vi "LS_SETP.vi"(8 "error in (no error)":errorcluster, 9 "Set Point (K)":dbl, 10 "Data Cluster In":T3 {"GUI Data Cluster"."SBR" format="%08b"}, 11 "Config Cluster In":T1={"General"={"Config.ini"=path "", "Default Logging Path"=path ""}, "Hardware"={"Measure Rate (1/s)"=0, "HP DMM VISA"="", "LS 335 VISA"="", "HP DM"={"Range"=enum."Autorange", "Autozero"=FALSE, "Display"=enum."3 1/2 Digit", "Blank LCD"=FALSE}, "LS335"={"Brightness"=enum."25%"}}, "Operation"={"Operation Mode"=enum."Logging", "Status"="", "NewLog?"=FALSE, "OvenWarn"=FALSE, "LS335"={"Heater A"={"Range"=enum."Off", "Set Point"=0.0}, "Heater B"={"Range"=enum."Off", "Set Point"=0.0}}}}) -> (0 "error out":errorcluster, 2 "Data Cluster Out":T3 {"GUI Data Cluster"."SBR" format="%08b"}, 3 "Config Cluster Out":T1={"General"={"Config.ini"=path "", "Default Logging Path"=path ""}, "Hardware"={"Measure Rate (1/s)"=0, "HP DMM VISA"="", "LS 335 VISA"="", "HP DM"={"Range"=enum."Autorange", "Autozero"=FALSE, "Display"=enum."3 1/2 Digit", "Blank LCD"=FALSE}, "LS335"={"Brightness"=enum."25%"}}, "Operation"={"Operation Mode"=enum."Idle-Off", "Status"="", "NewLog?"=FALSE, "OvenWarn"=FALSE, "LS335"={"Heater A"={"Range"=enum."Off", "Set Point"=0.0}, "Heater B"={"Range"=enum."Off", "Set Point"=0.0}}}}, 5 "return count":u32)   [LabVIEW 2021]
uses:
  Config_Cluster.ctl
  Mode_Enum.ctl
  Data_Cluster.ctl
  Measurement_Cluster.ctl
panel:
  in  "Heater":enum16{"A", "B"}(ring)
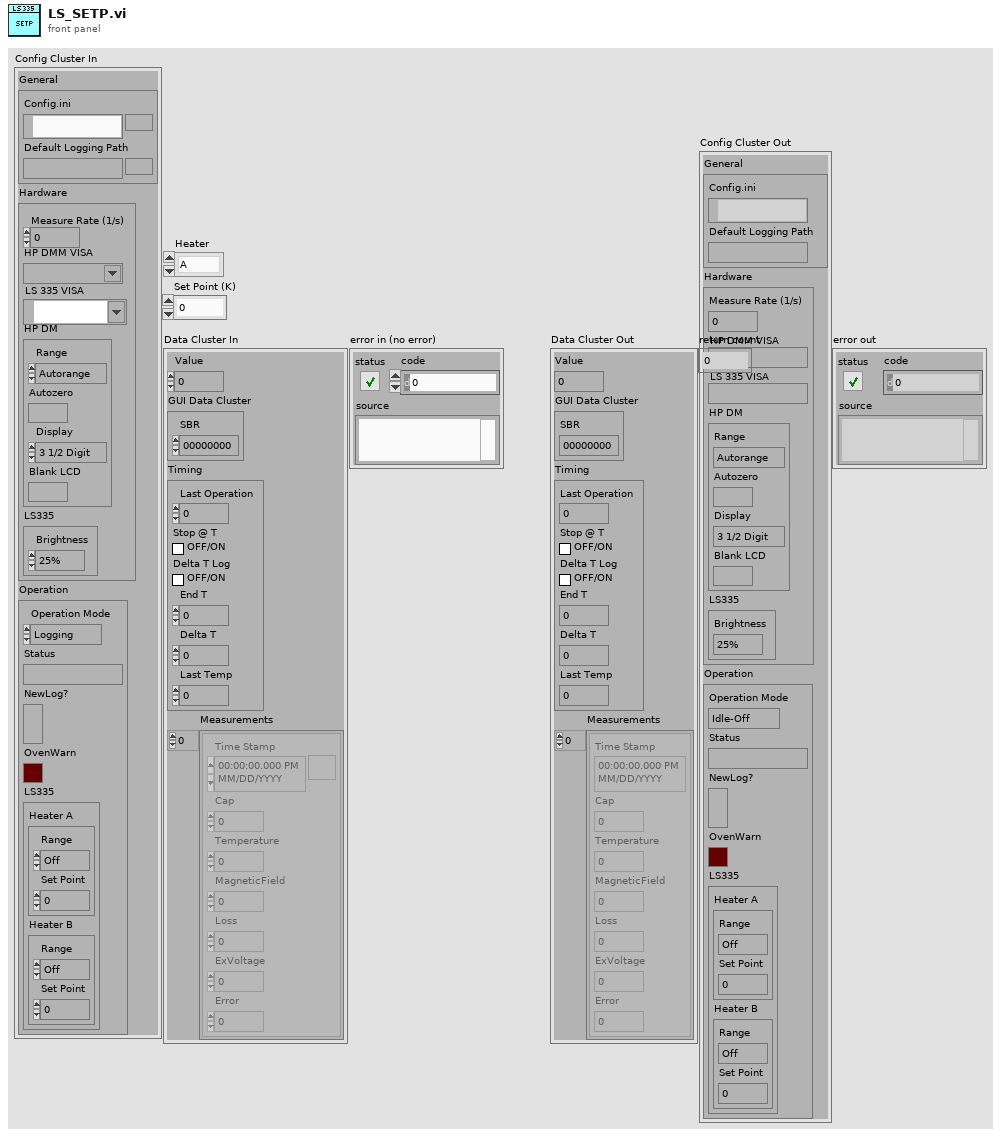
[diagram p1: front panel]
types:
  T1 = typedef "Config_Cluster.ctl" = cluster{"General":cluster{"Config.ini":path, "Default Logging Path":path}, "Hardware":cluster{"Measure Rate (1/s)":i32, "HP DMM VISA":refnum<visa-resource-name>, "LS 335 VISA":refnum<visa-resource-name>, "HP DM":cluster{"Range":enum16{"Autorange", "30mV", "300mV", "3V", "30V"}, "Autozero":bool, "Display":enum16{"3 1/2 Digit", "4 1/2 Digit", "5 1/2 Digit"}, "Blank LCD":bool}, "LS335":cluster{"Brightness":enum16{"25%", "50%", "75%", "100%"}}}, "Operation":cluster{"Operation Mode":T2, "Status":string, "NewLog?":bool, "OvenWarn":bool, "LS335":cluster{"Heater A":cluster{"Range":enum16{"Off", "Low", "Medium", "High"}, "Set Point":dbl}, "Heater B":cluster{"Range":enum16{"Off", "Low", "Medium", "High"}, "Set Point":dbl}}}}
  T2 = typedef "Mode_Enum.ctl" = enum16{"OvenNRDY", "Logging", "Idle-Off", "Idle"}
  T3 = typedef "Data_Cluster.ctl" = cluster{"Value":dbl, "GUI Data Cluster":cluster{"SBR":u16}, "Timing":cluster{"Last Operation":dbl, "Stop @ T":bool, "Delta T Log":bool, "End T":dbl, "Delta T":dbl, "Last Temp":dbl}, "Measurements":T4[]}
  T4 = typedef "Measurement_Cluster.ctl" = cluster{"Time Stamp":timestamp, "Cap":dbl, "Temperature":dbl, "MagneticField":dbl, "Loss":dbl, "ExVoltage":dbl, "Error":dbl}
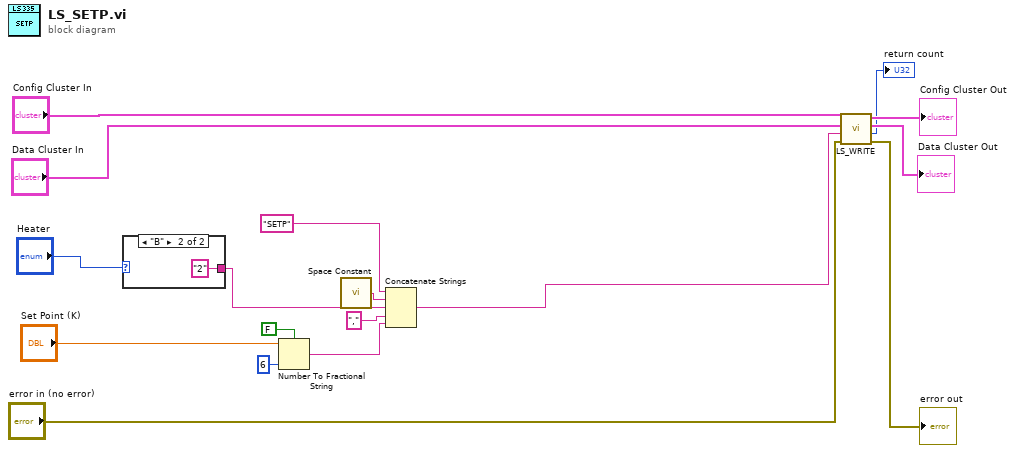
[diagram p0: block diagram]
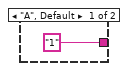
[diagram p2: hidden frame]
diagram:
  n1 = case shown="\"B\"" "Heater" {
    tunnel: ["1" "2"] -> w7
    frame "A", Default {
    }
    frame "B" {
    }
  }
  n2 = Number To Fractional String(use system decimal point (T)=FALSE, number="Set Point (K)", precision (6)=i16 6) -> (F-format string=w2:string)  [unwired: 1 in]
  n3 = call <vilib>:"Space Constant.vi"() -> ("String"=w8:string)
  n4 = Concatenate Strings("SETP", w8, w7, ",", w2) -> (w1:string)
  n5 = call "LS_WRITE.vi"("error in (no error)"="error in (no error)", "write buffer"=w1, "Data Cluster In"="Data Cluster In", "Config Cluster In"="Config Cluster In") -> ("error out"=→"error out":errorcluster, "return count"=→"return count":u32, "Data Cluster Out"=→"Data Cluster Out":T3, "Config Cluster Out"=→"Config Cluster Out":T1)  [unwired: 4 in]
